vi "Interpolate 2D Scattered_Wn1.vi"(0 "X(Tri) In":dbl[][](array[numeric]), 5 "Y(Tri) In":dbl[][](array[numeric]), 7 "Z(Tri) In":dbl[][](array[numeric]), 9 "gx in":dbl[][](array[numeric]), 11 "gy in":dbl[][](array[numeric]), 12 "Length":dbl[][](array[numeric])) -> (4 "X(Tri) Out":dbl[][](array[numeric]), 6 "Y(Tri) Out":dbl[][](array[numeric]), 8 "Z(Tri) Out":dbl[][](array[numeric]), 10 "gx out":dbl[][](array[numeric]), 14 "Wn 1":dbl[][](array[numeric]), 15 "gy out":dbl[][](array[numeric]))   [LabVIEW 2017, in "NI_AAL_Interpolation.lvlib"]
uses:
  <vilib>/gmath/NI_AAL_Interpolation.lvlib
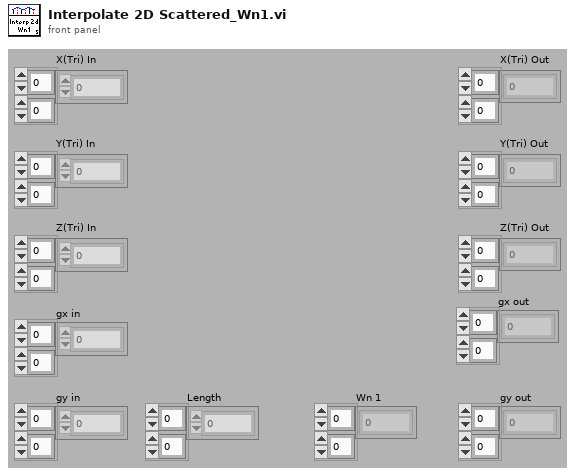
[diagram p1: front panel]
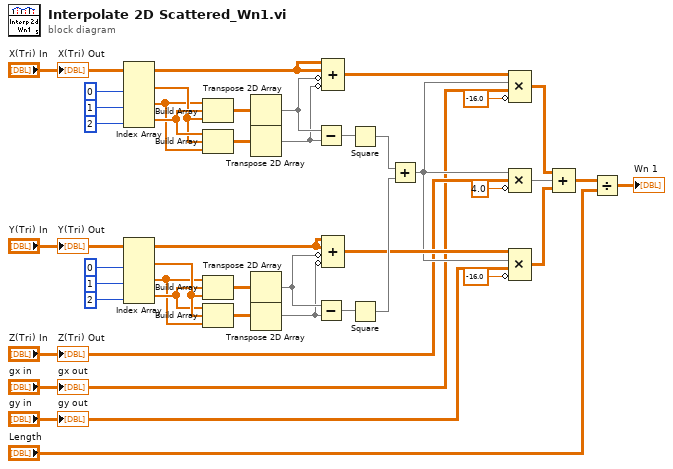
[diagram p0: block diagram]
diagram:
  n1 = Index Array(array="X(Tri) In", index (col) #1=0 ("disabled index (col)"), index (col) #2=1 ("index (col)"), index (col) #3=2 ("index (col)")) -> (element #1=w34:dbl[], element #2=w33:dbl[], element #3=w35:dbl[])  [unwired: 3 in]
  n2 = Index Array(array="Y(Tri) In", index (col) #1=0 ("disabled index (col)"), index (col) #2=1 ("index (col)"), index (col) #3=2 ("index (col)")) -> (element #1=w32:dbl[], element #2=w30:dbl[], element #3=w31:dbl[])  [unwired: 3 in]
  n3 = Build Array(w33, w35, w34) -> (w27:dbl[][])
  n4 = Build Array(w35, w34, w33) -> (w26:dbl[][])
  n5 = Build Array(w30, w31, w32) -> (w29:dbl[][])
  n6 = Build Array(w31, w32, w30) -> (w28:dbl[][])
  n7 = Transpose 2D Array(2D array=w27) -> (transposed array=w10:dbl[][])
  n8 = Transpose 2D Array(2D array=w26) -> (transposed array=w9:dbl[][])
  n9 = Transpose 2D Array(2D array=w29) -> (transposed array=w8:dbl[][])
  n10 = Transpose 2D Array(2D array=w28) -> (transposed array=w7:dbl[][])
  n11 = Subtract(x=w10, y=w9) -> (x-y=w23:dbl[][])
  n12 = Subtract(x=w8, y=w7) -> (x-y=w19:dbl[][])
  n13 = Compound Arithmetic op=ADD("X(Tri) In", "X(Tri) In", invert w10, invert w9) -> (w24:dbl[][])
  n14 = Compound Arithmetic op=ADD("Y(Tri) In", "Y(Tri) In", invert w8, invert w7) -> (w17:dbl[][])
  n15 = Square(x=w23) -> (x^2=w22:dbl[][])
  n16 = Square(x=w19) -> (x^2=w21:dbl[][])
  n17 = Add(x=w22, y=w21) -> (x+y=w16:dbl[][])
  n18 = Compound Arithmetic op=MULTIPLY(w24, w16, "gx in", invert -16.0) -> (w15:dbl[][])
  n19 = Compound Arithmetic op=MULTIPLY(w16, "Z(Tri) In", invert 4.0) -> (w14:dbl[][])
  n20 = Compound Arithmetic op=MULTIPLY(w17, w16, "gy in", invert -16.0) -> (w13:dbl[][])
  n21 = Compound Arithmetic op=ADD(w15, w14, w13) -> (w12:dbl[][])
  n22 = Divide(x=w12, y="Length") -> (x/y=→"Wn 1":dbl[][])
  "X(Tri) Out" <- "X(Tri) In"
  "Y(Tri) Out" <- "Y(Tri) In"
  "Z(Tri) Out" <- "Z(Tri) In"
  "gx out" <- "gx in"
  "gy out" <- "gy in"
